vi "Initialize.vi"(8 "error in (no error)":errorcluster, 9 "ID Query":bool, 10 "Reset":bool, 11 "Total Phase Aardvark in":refnum<class "Total Phase Aardvark.lvclass">) -> (0 "error out":errorcluster, 2 "VISA resource name":refnum<visa-resource-name>, 3 "Total Phase Aardvark out":refnum<class "Total Phase Aardvark.lvclass">)   [LabVIEW 2016, in "Host Adapter.lvlib" / "Total Phase Aardvark.lvlib" / "Total Phase Aardvark.lvclass"]
uses:
  Total Phase Aardvark.lvclass
panel:
  in  "Done":bool
  in  "Port":u16(ring) items=["0"]
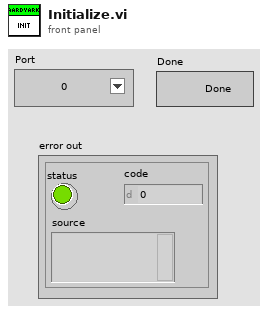
[diagram p1: front panel]
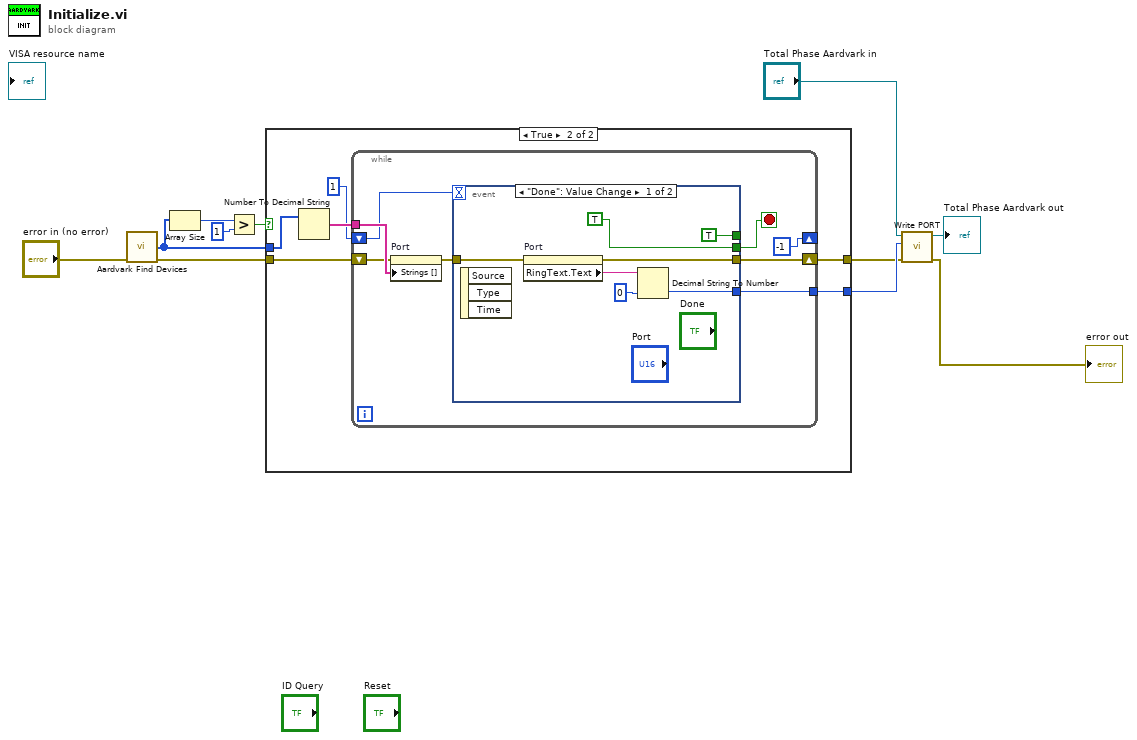
[diagram p0: block diagram]
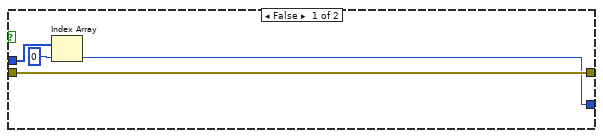
[diagram p2: hidden frame]
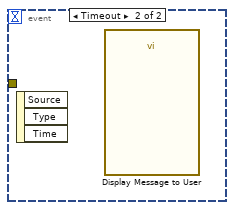
[diagram p3: hidden frame]
diagram:
  n1 = call <instrlib>:"Aardvark Find Devices.vi"("error in (no error)"="error in (no error)") -> ("Ports"=w8:u16[], "error out"=w4:errorcluster)  [unwired: 12 in, 1 out]
  n2 = Array Size(array=w8) -> (size(s)=w10:i32)
  n3 = Greater?(x=w10, y=1) -> (0:w2:bool)
  n4 = case shown="True" w2 {
    tunnel: w8 -> [w15 w21]
    tunnel: [w12 w19] -> w5
    tunnel: w4 -> [w13 w18]
    tunnel: [w13 w17] -> w3
    frame False {
      n5 = Index Array(array=w15, index=0) -> (element=w12:u16)
    }
    frame True {
      n6 = Number To Decimal String(number=w21) -> (decimal integer string=w20:string[])  [unwired: 1 in]
      n7 = while {
        tunnel: w20 -> [w29]
        tunnel: [w28] -> w19
        shift-right: [w25] -> w17
        shift-left: w18 -> [w27]
        shift-right: [-1] -> _
        shift-left: 1 -> [w23]
        stop <- w24 stop-if-true
        n8 = property on="Port" class="Ring (strict)"(error in=w27, "Strings []"=w29) -> (error out=w26:errorcluster)  [unwired: 1 in, 1 out]
        n9 = event shown="[0] \"Done\": Value Change" {
          selector: _ -> [_ _]
          dyn-events: _ -> [_ _]
          timeout: w23 -> [_ _]
          tunnel: [TRUE _] -> _
          tunnel: [w34 _] -> w28
          tunnel: w26 -> [w33 _]
          tunnel: [w32 _] -> w25
          tunnel: [TRUE _] -> w24
          event "Done": Value Change {
            n10 = event-data() -> ()  [unwired: 1 in, 3 out]
            n11 = property on="Port" class="Ring (strict)"(error in=w33) -> (error out=w32:errorcluster, "RingText.Text"=w35:string)  [unwired: 1 in, 1 out]
            n12 = Decimal String To Number(string=w35, default (0L)=u16 0 ("default (0 I32)")) -> (number=w34:u16)  [unwired: 1 in, 1 out]
          }
          event Timeout {
            n13 = event-data() -> ()  [unwired: 1 in, 3 out]
            n14 = call "Display Message to User"() -> ()  [unwired: 10 in, 2 out]
          }
        }
      }
    }
  }
  n15 = call-dynamic "Write PORT.vi"("error in (no error)"=w3, "PORT"=w5, "Host Adapter in"="Total Phase Aardvark in") -> ("error out"=→"error out":errorcluster, "Host Adapter out"=→"Total Phase Aardvark out":refnum<class "Total Phase Aardvark.lvclass">)  [unwired: 7 in]
